vi "PC_initialize_logging_file.vi"(8 "error in (no error)":errorcluster, 11 "Path":path) -> (0 "error out":errorcluster)   [LabVIEW 2020]
uses:
  output_headers.ctl
  <vilib>/Utility/file.llb/Write Delimited Spreadsheet (string).vi
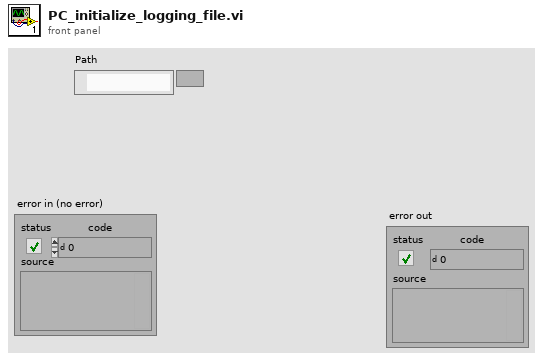
[diagram p1: front panel]
types:
  T1 = typedef "output_headers.ctl" = string[]
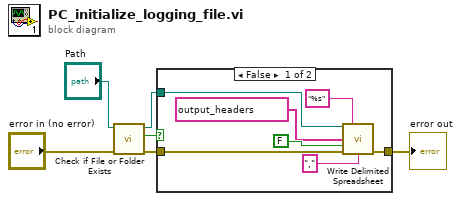
[diagram p0: block diagram]
diagram:
  n1 = call <vilib>:"Check if File or Folder Exists.vi"("error in (no error)"="error in (no error)", "path"="Path") -> ("error out"=w4:errorcluster, "file or folder exists?"=w5:bool, "dup path"=w1:path)  [unwired: 7 in]
  n2 = case shown="False" w5 {
    tunnel: w4 -> [w13 w14]
    tunnel: [w12 w14] -> w3
    tunnel: w1 -> [w8 _]
    frame False {
      n3 = call-poly <vilib>:"Write Delimited Spreadsheet.vi"("file path (dialog if empty)"=w8, "format (%s)"="%s" ("format (%.3f)"), "1D data"=T1 ["timestamp", "ac_freq", "ac_volt", "mod_type", "mod_waveform", "mod_freq", "mod_depth", "dio0", "dio1", "dio2", "dio3", "channel_enabled", "modulation_enabled"] ("Headers"), "append to file? (new file:F)"=FALSE, "error in (no error)"=w13, "delimiter (\\t)"="," ("delimiter (\\t)")) -> ("error out"=w12:errorcluster)  [unwired: 8 in, 1 out]
    }
    frame True {
    }
  }
  "error out" <- w3
